vi "Find Two Peaks (SubVI).vi"(7 "N Points":u16, 11 "Peak Index":u16[](array[numeric])=[0, 0, 0]) -> (0 "V2":u16, 3 "V1":u16)   [LabVIEW 2015]
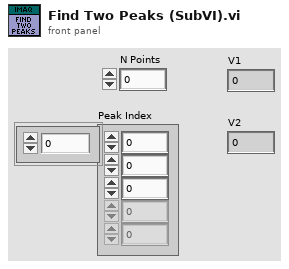
[diagram p1: front panel]
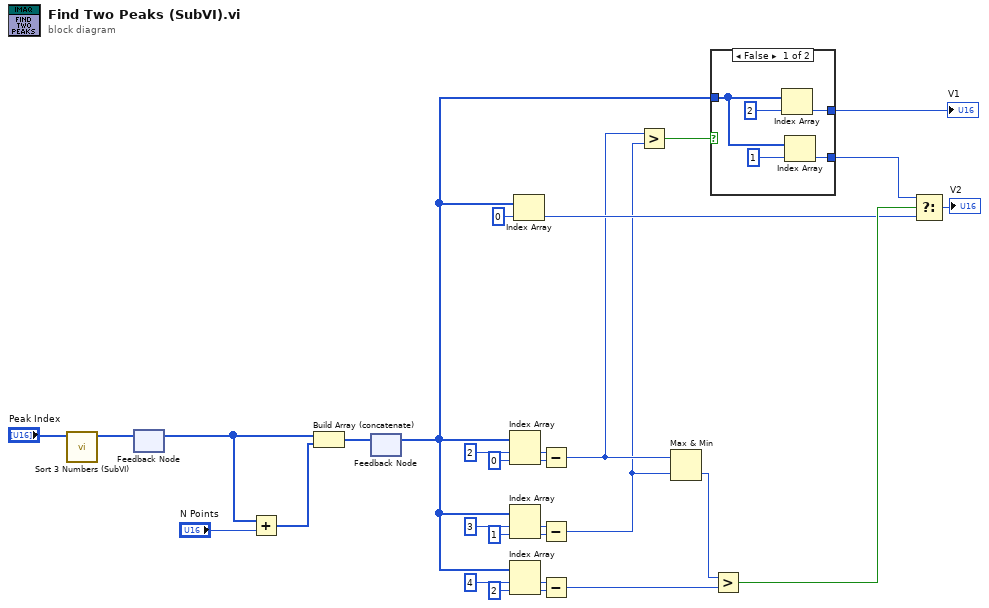
[diagram p0: block diagram]
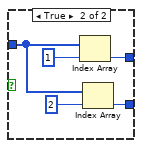
[diagram p2: hidden frame]
diagram:
  n1 = call "Sort 3 Numbers (SubVI).vi"("Array In"="Peak Index") -> ("Array Out"=w14:u16[])  [unwired: 10 in]
  n2 = feedback-in #1(w14) -> ()
  n3 = feedback #1() -> (w13:u16[])  [unwired: 1 in]
  n4 = Add(x=w13, y="N Points") -> (x+y=w15:u16[])
  n5 = Build Array (concatenate)(w13, w15) -> (w30:u16[])
  n6 = feedback #2() -> (w11:u16[])  [unwired: 1 in]
  n7 = feedback-in #2(w30) -> ()
  n8 = Index Array(array=w11, index #1=2 ("index"), index #2=0 ("index")) -> (element #1=w17:u16, element #2=w18:u16)
  n9 = Index Array(array=w11, index #1=3 ("index"), index #2=1 ("index")) -> (element #1=w24:u16, element #2=w23:u16)
  n10 = Index Array(array=w11, index #1=4 ("index"), index #2=2 ("index")) -> (element #1=w25:u16, element #2=w26:u16)
  n11 = Index Array(array=w11, index=0) -> (element=w5:u16)
  n12 = Subtract(x=w17, y=w18) -> (x-y=w4:u16)
  n13 = Subtract(x=w24, y=w23) -> (x-y=w3:u16)
  n14 = Subtract(x=w25, y=w26) -> (x-y=w2:u16)
  n15 = Greater?(x=w4, y=w3) -> (0:w12:bool)
  n16 = Max & Min(x=w4, y=w3) -> (min(x,y)=w7:u16)  [unwired: 1 out]
  n17 = case shown="False" w12 {
    tunnel: w11 -> [w31 w36]
    tunnel: [w34 w39] -> w10
    tunnel: [w32 w37] -> w8
    frame False {
      n18 = Index Array(array=w31, index=2) -> (element=w34:u16)
      n19 = Index Array(array=w31, index=1) -> (element=w32:u16)
    }
    frame True {
      n20 = Index Array(array=w36, index=1) -> (element=w39:u16)
      n21 = Index Array(array=w36, index=2) -> (element=w37:u16)
    }
  }
  "V1" <- w10
  n22 = Greater?(x=w7, y=w2) -> (0:w9:bool)
  n23 = Select(t=w8, s=w9, f=w5) -> (s? t:f=→"V2":u16)
